vi "Get All Endpoints.vi"(8 "error in (no error)":errorcluster, 11 "Aliases Ref in":T1 format="%.0x") -> (0 "error out":errorcluster, 2 "Addressable Endpoints":cluster{"Module":string, "Endpoint":string}[](array[cluster]), 3 "Aliases Ref out":T1 format="%.0x")   [LabVIEW 2020, in "Routing and Faulting System Explorer.lvlib"]
uses:
  Routing and Faulting System Explorer.lvlib
  <vilib>/NI VeriStand/Custom Device API/Custom Device Item Ref.ctl
  <vilib>/NI VeriStand/Custom Device API/Custom Device API.lvlib
  Shared/Routing and Faulting Hardware API/Routing and Faulting Hardware API.lvlib
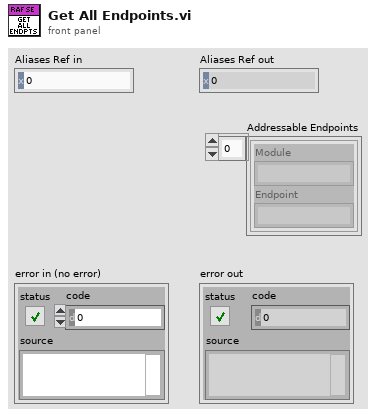
[diagram p1: front panel]
types:
  T1 = typedef "Custom Device API.lvlib/Custom Device Item Ref.ctl" = u64
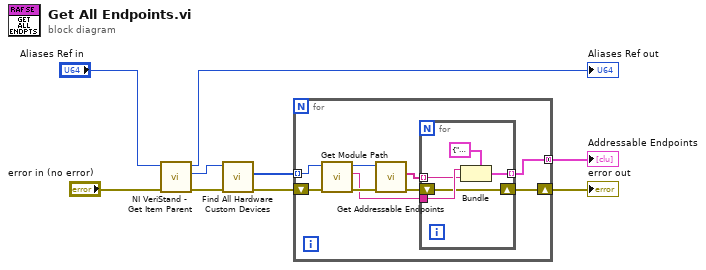
[diagram p0: block diagram]
diagram:
  n1 = call <vilib>:"NI VeriStand - Get Item Parent.vi"("error in (no error)"="error in (no error)", "Item Ref in"="Aliases Ref in") -> ("error out"=w7:errorcluster, "Parent Ref"=w6:T1, "Item Ref out"=→"Aliases Ref out":T1)  [unwired: 6 in, 1 out]
  n2 = call "Find All Hardware Custom Devices.vi"("error in (no error)"=w7, "Routing and Faulting Ref in"=w6) -> ("error out"=w4:errorcluster, "Hardware Refs"=w5:T1[])  [unwired: 7 in, 1 out]
  n3 = for {
    tunnel: w5 -> [w17] mode=indexing
    shift-right: [w13] -> w3
    shift-left: w4 -> [w18]
    tunnel: [w10] -> w1 mode=concatenating
    n4 = call "Get Module Path.vi"("error in (no error)"=w18, "Hardware Ref in"=w17) -> ("error out"=w15:errorcluster, "Module Path"=w11:string, "Hardware Ref out"=w16:T1)  [unwired: 6 in, 1 out]
    n5 = call "Get Addressable Endpoints.vi"("error in (no error)"=w15, "Hardware Ref in"=w16) -> ("error out"=w14:errorcluster, "Addressable Endpoints"=w12:string[])  [unwired: 6 in, 2 out]
    n6 = for {
      shift-right: [w21] -> w13
      shift-left: w14 -> [w21]
      tunnel: w12 -> [w22] mode=indexing
      tunnel: w11 -> [w23]
      tunnel: [w20] -> w10 mode=indexing
      n7 = Bundle(cluster=cluster{"Module":string, "Endpoint":string} {"Module"="", "Endpoint"=""}, "Module"=w23, "Endpoint"=w22) -> (w20:cluster{"Module":string, "Endpoint":string})
    }
  }
  "error out" <- w3
  "Addressable Endpoints" <- w1
